vi "CurrentTimeString.vi"() -> (3 "date/time string":string)   [LabVIEW 2013, in "main.lvlib"]
uses:
  main.lvlib
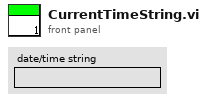
[diagram p1: front panel]
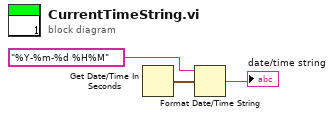
[diagram p0: block diagram]
diagram:
  n1 = Get Date/Time In Seconds() -> (seconds since 1Jan1904=w1:timestamp)
  n2 = Format Date/Time String(time format string (%c)="%Y-%m-%d %H%M", seconds (now)=w1) -> (date/time string=→"date/time string":string)  [unwired: 1 in]
